vi "checkSoakTimeElapsed.vi"(8 "error in (no error)":errorcluster, 11 "TestMonitor in":refnum<class "TestMonitor.lvclass">) -> (0 "error out":errorcluster, 1 "Wait Time Status":T1 {"Time Remaining" min=1.0 format="%.1f"}, 2 "soakTimeElapsedIsTrue":bool, 3 "TestMonitor out":refnum<class "TestMonitor.lvclass">)   [LabVIEW 2013, in "TestMonitor.lvclass"]
uses:
  TestMonitor.lvclass
  Typedefs/WaitTimeStatus.ctl
  TestMonitor.lvclass/TestMonitor.ctl
  Typedefs/AITDTTypedefs.lvlib
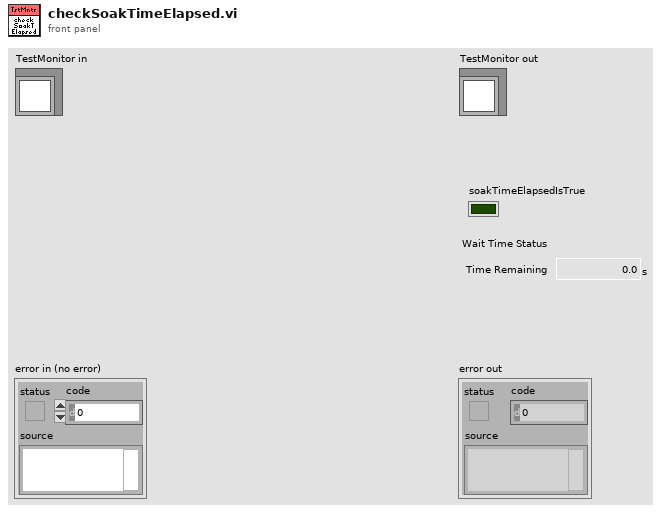
[diagram p1: front panel]
types:
  T1 = typedef "AITDTTypedefs.lvlib/WaitTimeStatus.ctl" = cluster{"Time Remaining":dbl[unit]}
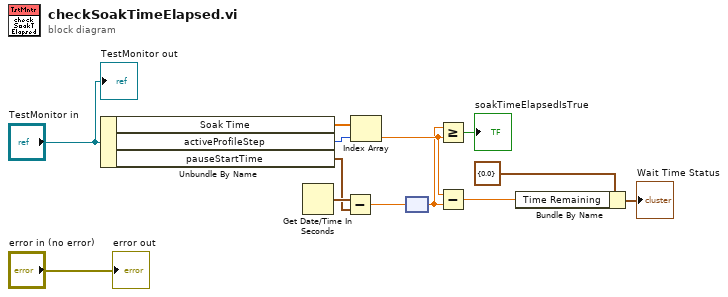
[diagram p0: block diagram]
diagram:
  n1 = Unbundle By Name("TestMonitor in") -> ("Soak Time"=w9:dbl[unit][], "activeProfileStep"=w8:u32, "pauseStartTime"=w10:timestamp)
  n2 = Get Date/Time In Seconds() -> (seconds since 1Jan1904=w11:timestamp)
  n3 = Subtract(x=w11, y=w10) -> (x-y=w7:dbl)
  n4 = Index Array(array=w9, index=w8) -> (element=w2:dbl[unit])
  n5 = node(w7) -> (w1:dbl[unit])
  n6 = Greater Or Equal?(x=w1, y=w2) -> (x >= y?=→"soakTimeElapsedIsTrue":bool)
  n7 = Subtract(x=w2, y=w1) -> (x-y=w3:dbl[unit])
  n8 = Bundle By Name(cluster=T1 {"Time Remaining"=0.0} ("Wait Time Status"), "Time Remaining"=w3) -> (→"Wait Time Status":T1)
  "error out" <- "error in (no error)"
  "TestMonitor out" <- "TestMonitor in"
